vi "Read.vi"(8 "error in (no error)":errorcluster, 11 "String in":refnum<class "Const_Str.lvclass">) -> (0 "error out":errorcluster, 2 "String":string, 3 "String out":refnum<class "Const_Str.lvclass">)   [LabVIEW 2021, in "Const_Str.lvclass"]
uses:
  Const_Str.lvclass
  Const_Str.lvclass/Const_Str.ctl
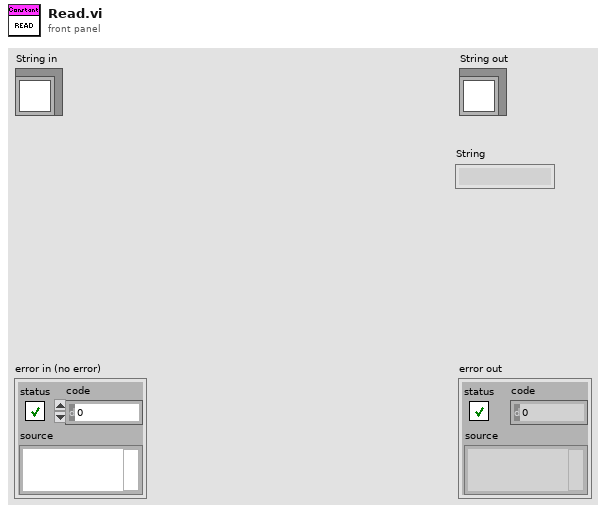
[diagram p1: front panel]
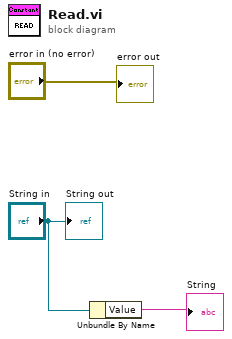
[diagram p0: block diagram]
diagram:
  n1 = Unbundle By Name("String in") -> ("Value"=→"String":string)
  "error out" <- "error in (no error)"
  "String out" <- "String in"
